vi "ReadObject.vi"(8 "Error In":errorcluster, 11 "object in":refnum<class "ObjectDecorator.lvclass">) -> (0 "Error Out":errorcluster, 2 "Object":refnum<class "Object.lvclass">, 3 "object out":refnum<class "ObjectDecorator.lvclass">)   [LabVIEW 2020, in "ObjectDecorator.lvclass"]
uses:
  ObjectDecorator.lvclass
  ObjectDecorator.lvclass/ObjectDecorator.ctl
  Object_interface/Object.lvclass
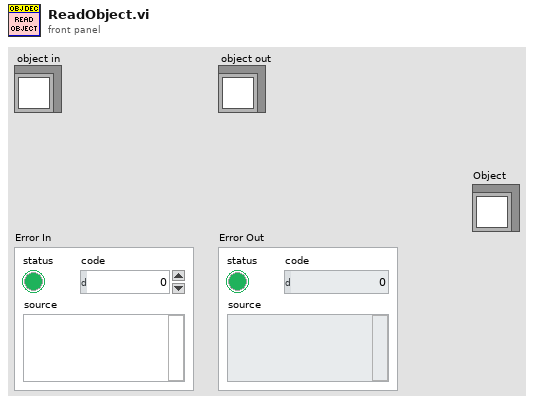
[diagram p1: front panel]
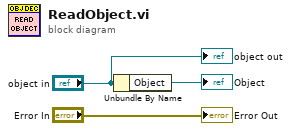
[diagram p0: block diagram]
diagram:
  n1 = Unbundle By Name("object in") -> ("Object"=→"Object":refnum<class "Object.lvclass">)
  "Error Out" <- "Error In"
  "object out" <- "object in"
